vi "Trigger_Coincidence_Logic.vi"(7 "Peak_ch1":dbl, 9 "Peak_ch4":dbl, 10 "Peak_ch3":dbl, 11 "Peak_ch2":dbl) -> (3 "Filter-out":bool)   [LabVIEW 2019]
uses:
  SiPM_Tests_Global_Var.vi
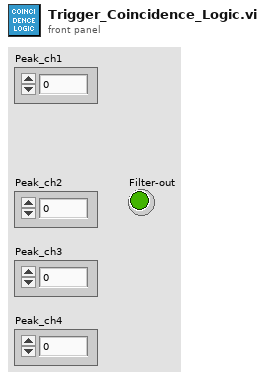
[diagram p1: front panel]
types:
  T1 = enum16{"Coincidence", "Anti-Coincidence", "Don't Care"}
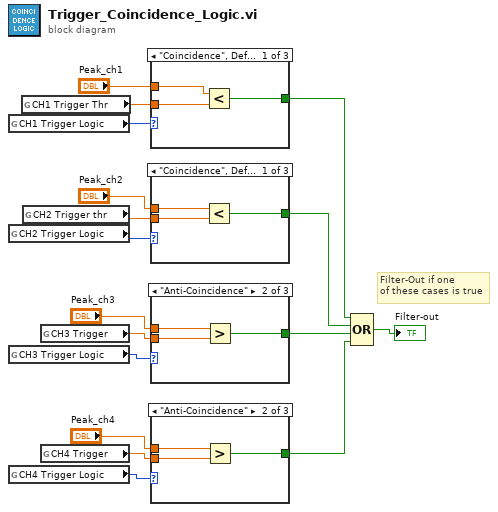
[diagram p0: block diagram]
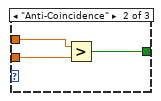
[diagram p2: hidden frame]
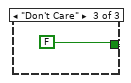
[diagram p3: hidden frame]
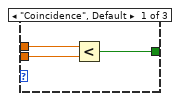
[diagram p4: hidden frame]
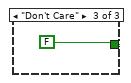
[diagram p5: hidden frame]
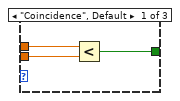
[diagram p6: hidden frame]
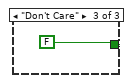
[diagram p7: hidden frame]
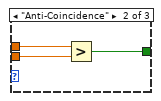
[diagram p8: hidden frame]
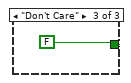
[diagram p9: hidden frame]
diagram:
  # "Filter-Out if one \nof these cases is true"
  n1 = global read "SiPM_Tests_Global_Var.vi" "CH1 Trigger Logic"() -> (w4:T1)
  n2 = global read "SiPM_Tests_Global_Var.vi" "CH2 Trigger Logic"() -> (w5:T1)
  n3 = global read "SiPM_Tests_Global_Var.vi" "CH3 Trigger Logic"() -> (w9:T1)
  n4 = global read "SiPM_Tests_Global_Var.vi" "CH4 Trigger Logic"() -> (w12:T1)
  n5 = global read "SiPM_Tests_Global_Var.vi" "CH1 Trigger Thr"() -> (w3:dbl)
  n6 = global read "SiPM_Tests_Global_Var.vi" "CH2 Trigger thr"() -> (w6:dbl)
  n7 = global read "SiPM_Tests_Global_Var.vi" "CH3 Trigger"() -> (w8:dbl)
  n8 = global read "SiPM_Tests_Global_Var.vi" "CH4 Trigger"() -> (w13:dbl)
  n9 = case shown="\"Coincidence\", Default" w4 {
    tunnel: [w20 w23 FALSE] -> w1
    tunnel: w3 -> [w19 w22 _]
    tunnel: "Peak_ch1" -> [w18 w21 _]
    frame "Coincidence", Default {
      n10 = Less?(x=w18, y=w19) -> (x < y?=w20:bool)
    }
    frame "Anti-Coincidence" {
      n11 = Greater?(x=w21, y=w22) -> (0:w23:bool)
    }
    frame "Don't Care" {
    }
  }
  n12 = case shown="\"Coincidence\", Default" w5 {
    tunnel: [w25 w28 FALSE] -> w14
    tunnel: w6 -> [w27 w29 _]
    tunnel: "Peak_ch2" -> [w26 w30 _]
    frame "Coincidence", Default {
      n13 = Less?(x=w26, y=w27) -> (x < y?=w25:bool)
    }
    frame "Anti-Coincidence" {
      n14 = Greater?(x=w30, y=w29) -> (0:w28:bool)
    }
    frame "Don't Care" {
    }
  }
  n15 = case shown="\"Anti-Coincidence\"" w9 {
    tunnel: [w32 w35 FALSE] -> w15
    tunnel: w8 -> [w34 w36 _]
    tunnel: "Peak_ch3" -> [w33 w37 _]
    frame "Coincidence", Default {
      n16 = Less?(x=w33, y=w34) -> (x < y?=w32:bool)
    }
    frame "Anti-Coincidence" {
      n17 = Greater?(x=w37, y=w36) -> (0:w35:bool)
    }
    frame "Don't Care" {
    }
  }
  n18 = case shown="\"Anti-Coincidence\"" w12 {
    tunnel: [w39 w42 FALSE] -> w16
    tunnel: w13 -> [w41 w43 _]
    tunnel: "Peak_ch4" -> [w40 w44 _]
    frame "Coincidence", Default {
      n19 = Less?(x=w40, y=w41) -> (x < y?=w39:bool)
    }
    frame "Anti-Coincidence" {
      n20 = Greater?(x=w44, y=w43) -> (0:w42:bool)
    }
    frame "Don't Care" {
    }
  }
  n21 = Compound Arithmetic op=OR(w1, w14, w15, w16) -> (→"Filter-out":bool)
